vi "niRFUtil RFHS Benchmark Start.vi"(11 "error in (no error)":errorcluster) -> (4 "Start Time":u64, 15 "error out":errorcluster)   [LabVIEW 2015, in "niRFUtil.lvlib"]
uses:
  niRFUtil.lvlib
  niRFUtil RFHS Util Phases.ctl
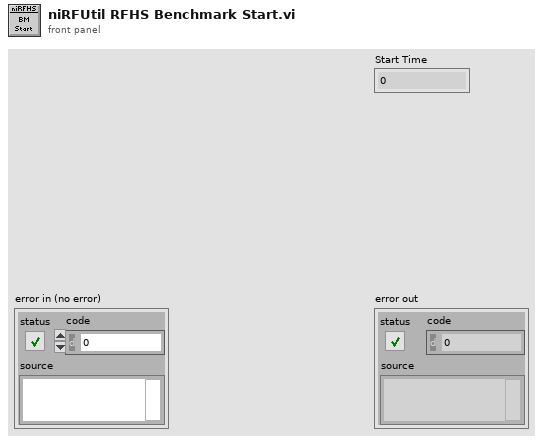
[diagram p1: front panel]
types:
  T1 = typedef "niRFUtil.lvlib/niRFUtil RFHS Util Phases.ctl" = enum32{"Reserved", "CreateBenchmarkTask", "CRC", "UE UL Segment Transport Block", "UE UL Read Buffer", "UE UL TC", "UE UL RM", "UE UL CI", "Scramble", "Group Bits", "Benchmark Task Start", "Benchmark Task Stop", "Descramble", "Deinterleave", "eNB UL HARQ", "eNB UL Read Buffer", "eNB UL AFEM", "eNB UL Turbo Decoder", "Get Benchmark Task Data", "G31", "UL Gen Freq2Time", "Gen Power Spectrum", "UL Ana Time2Freq", "Benchmark Task Enter", "Benchmark Task Leave"}
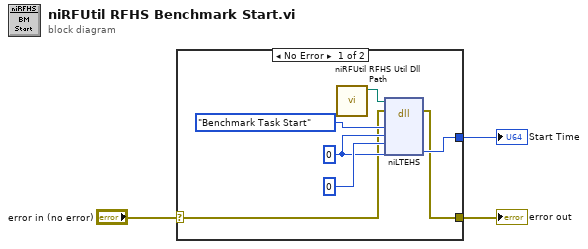
[diagram p0: block diagram]
diagram:
  n1 = case shown="No Error" "error in (no error)" {
    selector: "error in (no error)" -> [w5 w11]
    tunnel: [w4 w11] -> w2
    tunnel: [w6 _] -> w1
    frame No Error {
      w7 = u64 0 ("benchmarkTask")
      n2 = call "niRFUtil RFHS Util Dll Path.vi"() -> ("Path"=w10:path)  [unwired: 7 in, 4 out]
      n3 = dll-call lib="?" fn="niLTEHS"(path in=w10, error in=w5, "what"=niRFUtil_RFHS_Util_Phases."Benchmark Task Start" ("Enum"), "benchmarkTask"=w7, "benchId"=u32 0, "startTime"=w7) -> (error out=w4:errorcluster, "startTime"=w6:u64)  [unwired: 5 in, 1 out]
    }
    frame Error {
    }
  }
  "error out" <- w2
  "Start Time" <- w1
